vi "done(with var with tabs)subvi2backup.vi"(3 "error in (no error)":errorcluster, 5 "Image Src":T1) -> (0 "error out 2":errorcluster, 2 "Image Out 6":T1(plugin-control))   [LabVIEW 2011]
uses:
  <vilib>/vision/Image Controls.llb/IMAQ Image.ctl
  <vilib>/vision/NI_Vision_Development_Module.lvlib
panel:
  out "Image Dst Out":T1
  in  "Tab Control":T2(tab)
  out "Image Out 2":T1(plugin-control)
  out "Image Out 3":T1(plugin-control)
  out "Image Out 4":T1(plugin-control)
  out "Image Out 5":T1(plugin-control)
  out "Image Out 7":T1(plugin-control)
  in  "Parameters (OCR/OCV 1)":T3={"Threshold Mode"=1, "Fixed Threshold Range"={"Lower value"=1.0, "Upper value"=255.0}, "Advanced Threshold Data"={"Number of Blocks"=4, "Pixel Value Range"={"Lower value"=0, "Upper value"=255}, "Optimize For Speed"=FALSE, "Perform Bi-modal Calculation"=FALSE}, "Character Color"=0, "Reject Border"=FALSE, "Number Of Erosions"=0, "Size & Spacing"={"AutoSplit"=FALSE, "Min Bounding Rect Width"=160, "Max Bounding Rect Width"=200, "Min Bounding Rect Height"=200, "Max Bounding Rect Height"=240, "Min Character Size"=20, "Max Character Size"=65536, "Min Char Spacing"=1, "Max Horiz Element Spacing"=1, "Max Vert Element Spacing"=0}, "Read Options"={"Read Strategy"=1, "Read Resolution"=0, "Scale Dependant"=FALSE, "Aspect Ratio"=400, "Acceptance Level"=700, "Substitution Character"="?"}, "Valid Characters"=[], "Use Text Pattern"=FALSE, "Orientation"=0} {"Threshold Mode" items=["Fixed Range", "Uniform", "Linear", "Non Linear"]; "Character Color" items=["Dark on Light", "Light on Dark"]; "Read Options"."Read Strategy" items=["Aggressive", "Conservative"]; "Read Options"."Read Resolution" items=["Low", "Medium", "High"]; "Valid Characters"."Pre-defined characters" items=["Any Character", "User-defined Characters", "Alphabetic", "Alphanumeric", "Uppercase Letters", "Lowercase Letters", "Decimal Digits", "Hexadecimal Digits", "Pattern", "Force Space"]; "Orientation" items=["Baseline inside", "Baseline outside"]}
  in  "File Path (OCR/OCV 1)":path=path "D:/Program Files/National Instruments/Vision/OCR/CharacterSetFiles/OCRA30.abc"
  in  "ROI Descriptor (OCR/OCV 1)":T4={"Global Rectangle"=[390, 669, 561, 882], "Contours"=[{"ID"=enum."External", "Type"=3, "Coordinates"=[390, 669, 561, 882]}]} {"Contours"."Type" items=["No Selection", "Point", "Line", "Rectangle", "Oval", "Polygon", "Freehand Region", "Annulus", "Unused2", "Unused3", "Broken Line", "Freehand Line", "Rotated Rectangle"]}
  in  "Method (Filters 1)":T5(ring)=enum."Prewitt"
  in  "Niblack Deviation Factor (Threshold 1)":dbl=0.2
  in  "Kernel Size (Threshold 1)":cluster{"SizeX":i32, "SizeY":i32}={"SizeX"=32, "SizeY"=32}
  in  "Look For (Bright Objects) (Threshold 1)":u32(ring) items=["Bright Objects", "Dark Objects"]
  in  "Method (Threshold 1)":u32(ring)=1 items=["Niblack", "Background Correction"]
  in  "Color Plane (Color Plane Extraction 1)":i32(ring)=5 items=["Red", "Green", "Blue", "Hue", "Saturation", "Luminance", "Value", "Intensity"]
  out "String (OCR/OCV 1)":string
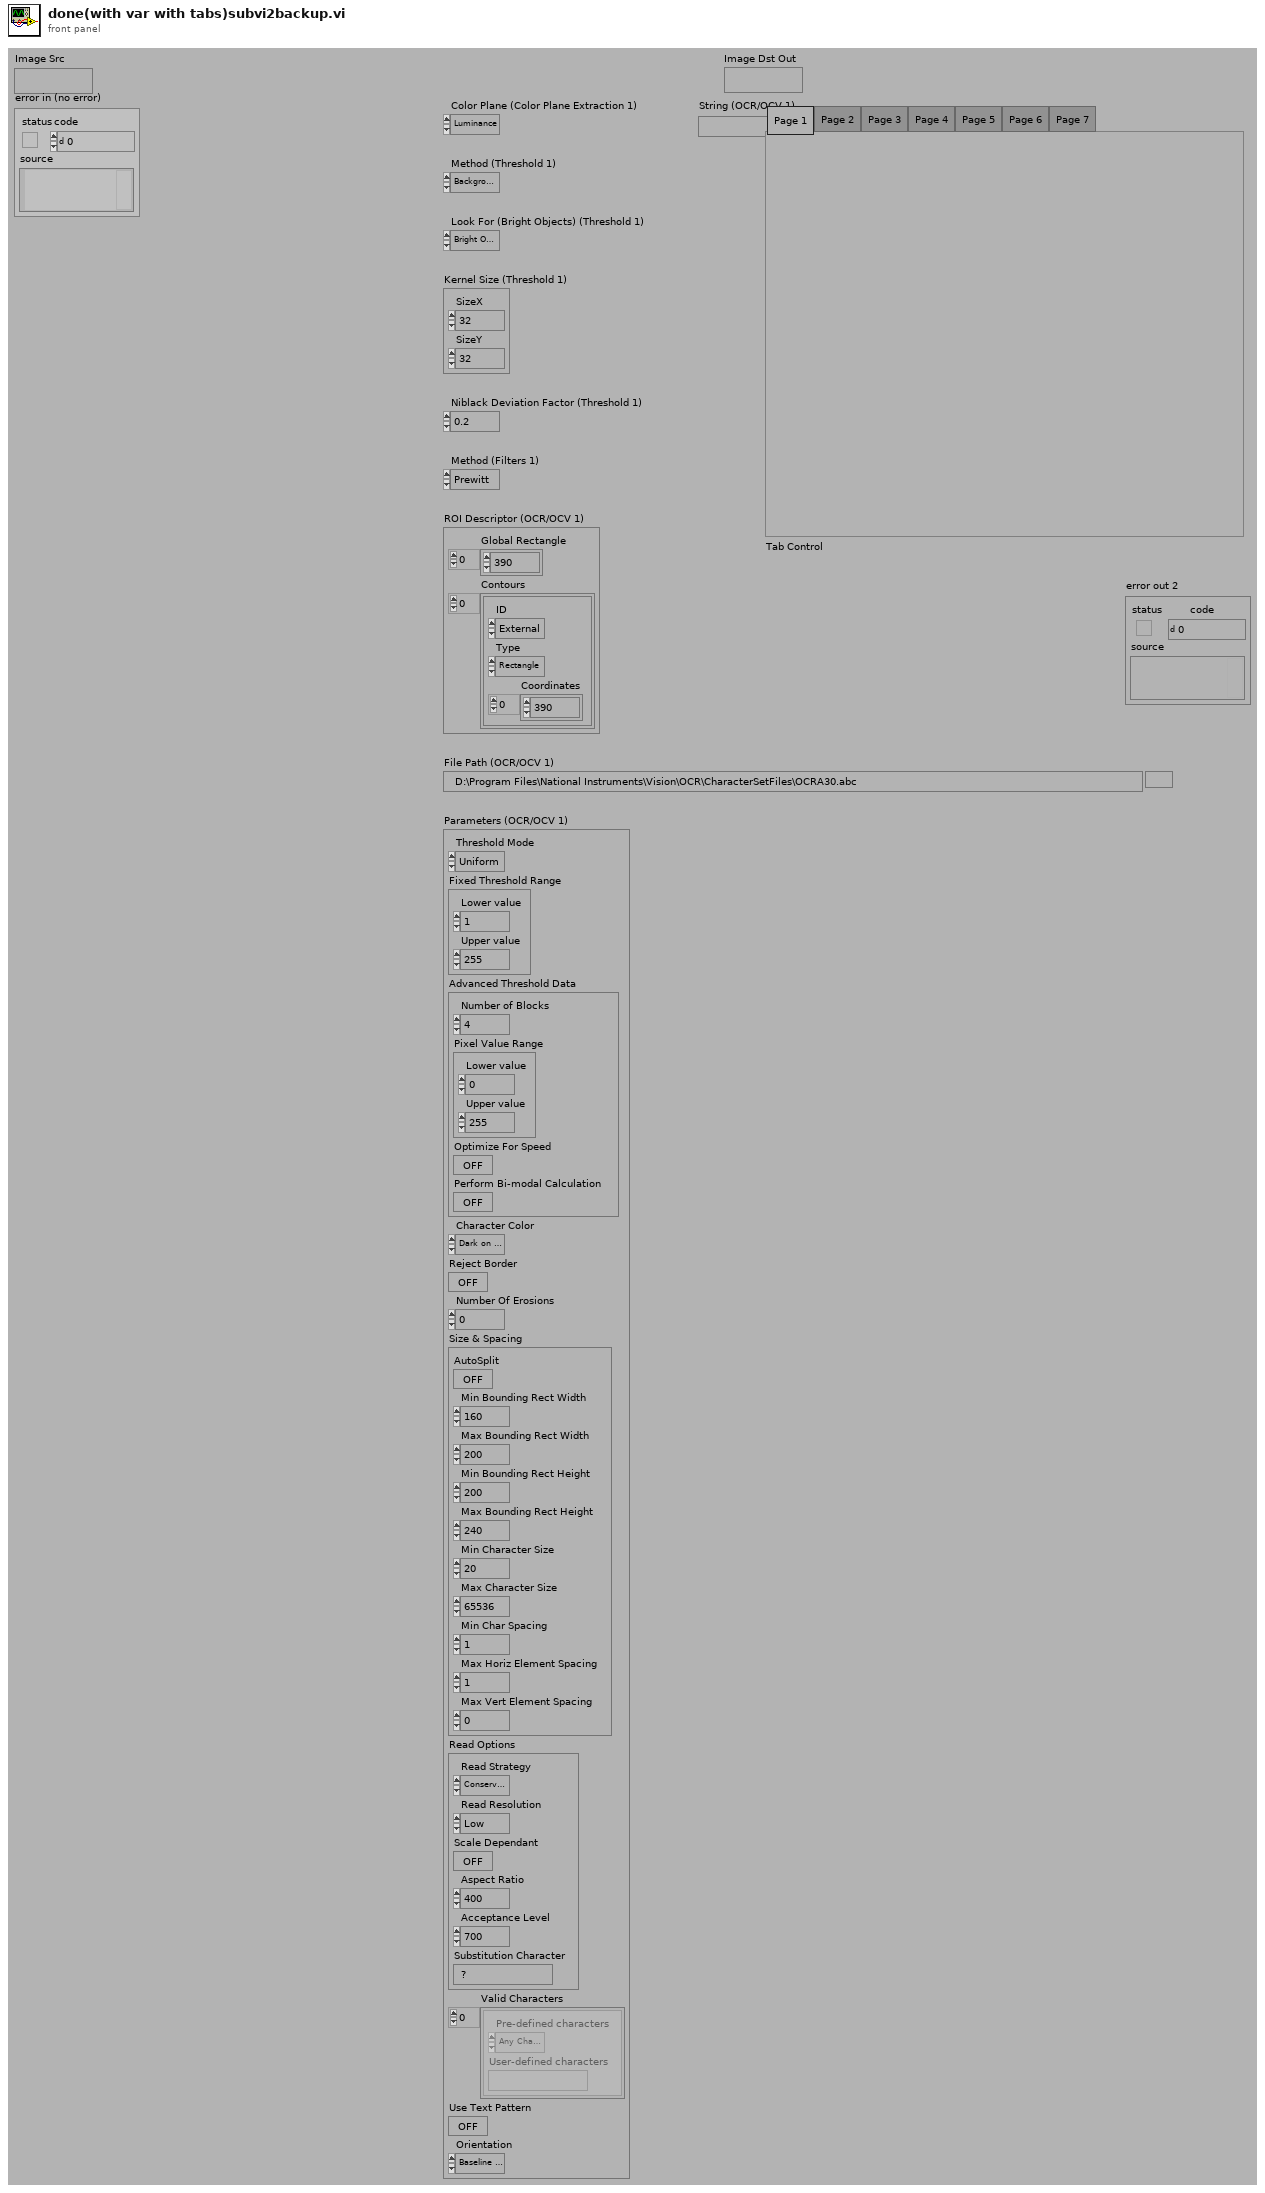
[diagram p1: front panel]
types:
  T1 = typedef "IMAQ Image.ctl" = refnum<image>
  T2 = enum32{"Page 1", "Page 2", "Page 3", "Page 4", "Page 5", "Page 6", "Page 7"}
  T3 = cluster{"Threshold Mode":i32, "Fixed Threshold Range":cluster{"Lower value":sgl, "Upper value":sgl}, "Advanced Threshold Data":cluster{"Number of Blocks":i32, "Pixel Value Range":cluster{"Lower value":i32, "Upper value":i32}, "Optimize For Speed":bool, "Perform Bi-modal Calculation":bool}, "Character Color":i32, "Reject Border":bool, "Number Of Erosions":i32, "Size & Spacing":cluster{"AutoSplit":bool, "Min Bounding Rect Width":i32, "Max Bounding Rect Width":i32, "Min Bounding Rect Height":i32, "Max Bounding Rect Height":i32, "Min Character Size":i32, "Max Character Size":i32, "Min Char Spacing":i32, "Max Horiz Element Spacing":i32, "Max Vert Element Spacing":i32}, "Read Options":cluster{"Read Strategy":i32, "Read Resolution":i32, "Scale Dependant":bool, "Aspect Ratio":i32, "Acceptance Level":i32, "Substitution Character":string}, "Valid Characters":cluster{"Pre-defined characters":i32, "User-defined characters":string}[], "Use Text Pattern":bool, "Orientation":u32}
  T4 = cluster{"Global Rectangle":i32[], "Contours":cluster{"ID":enum32{"External", "Internal"}, "Type":u32, "Coordinates":i32[]}[]}
  T5 = enum32{"Differentiation", "Gradient", "Prewitt", "Roberts", "Sigma", "Sobel"}
  T6 = cluster{"histogram":u32[], "Minimal Value":sgl, "Maximal Value":sgl, "Starting Value":sgl, "Interval Width":sgl, "Mean Value":sgl, "Standard  Variation":sgl, "Area (pixels)":i32}
  T7 = typedef "Image Type" = u32
  T8 = typedef "IMAQ OCR Session.ctl" = refnum<k1>
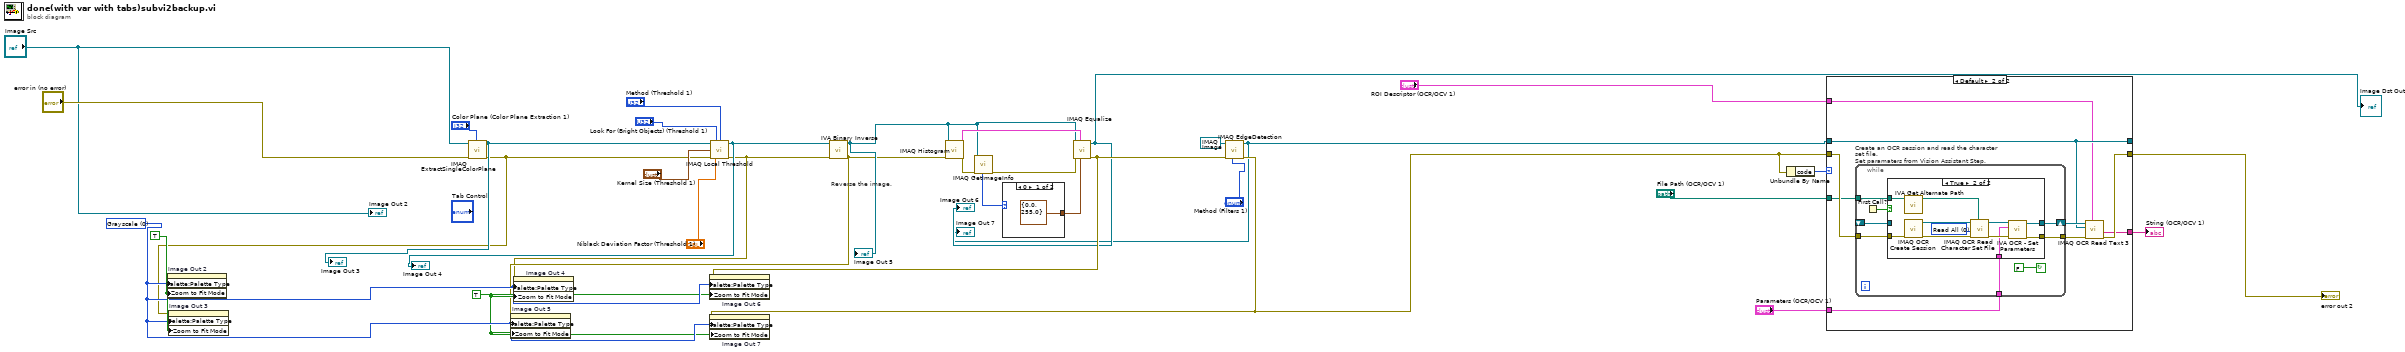
[diagram p0: block diagram]
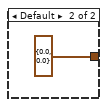
[diagram p4: hidden frame]
diagram:
  w16 = TRUE ("Zoom to Fit Mode")
  w18 = TRUE ("Zoom to Fit Mode")
  w17 = u32 0 items=["Grayscale", "Binary", "Gradient", "Rainbow", "Temperature", "User Defined"] ("Palette")
  # "Reverse the image."
  n1 = property on="Image Out 2" class="ImageControl"("Palette:Palette Type"=w17, "Zoom to Fit Mode"=w18) -> ()  [unwired: 2 in, 2 out]
  n2 = call "IMAQ ExtractSingleColorPlane"("Color Plane"="Color Plane (Color Plane Extraction 1)", "error in (no error)"="error in (no error)", "Image Src"="Image Src") -> ("error out"=w6:errorcluster, "Image Dst Out"=w14:T1)  [unwired: 1 in, 6 out]
  "Image Out 3" <- w14
  n3 = property on="Image Out 3" class="ImageControl"(error in=w6, "Palette:Palette Type"=w17, "Zoom to Fit Mode"=w18) -> ()  [unwired: 1 in, 2 out]
  n4 = call "IMAQ Local Threshold"("Image Src"=w14, "Look For (Bright Objects)"="Look For (Bright Objects) (Threshold 1)", "Method (Niblack)"="Method (Threshold 1)", "Window Size (32x32)"="Kernel Size (Threshold 1)", "error in (no error)"=w6, "Niblack Deviation Factor (0.2)"="Niblack Deviation Factor (Threshold 1)") -> ("Image Dst Out"=w13:T1, "error out"=w7:errorcluster)  [unwired: 2 in, 6 out]
  "Image Out 4" <- w13
  n5 = property on="Image Out 4" class="ImageControl"(error in=w7, "Palette:Palette Type"=w17, "Zoom to Fit Mode"=w16) -> ()  [unwired: 1 in, 2 out]
  n6 = call <vilib>:"IVA Binary Inverse.vi"("error in (no error)"=w7, "Image In"=w13) -> ("error out"=w8:errorcluster, "Image Out"=w12:T1)  [unwired: 8 out]
  "Image Out 5" <- w12
  n7 = property on="Image Out 5" class="ImageControl"(error in=w8, "Palette:Palette Type"=w17, "Zoom to Fit Mode"=w16) -> ()  [unwired: 1 in, 2 out]
  n8 = call "IMAQ Histogram"("error in (no error)"=w8, "Image"=w12) -> ("error out"=w15:errorcluster, "Histogram Report"=w28:T6)  [unwired: 3 in, 5 out]
  n9 = call "IMAQ GetImageInfo"("error in (no error)"=w15, "Image"=w12) -> ("error out"=w26:errorcluster, "Image Type"=w27:T7)  [unwired: 8 out]
  n10 = case shown="0" w27 {
    tunnel: [cluster{"Minimum":sgl, "Maximum":sgl} {"Minimum"=0.0, "Maximum"=255.0} ("Range") cluster{"Minimum":sgl, "Maximum":sgl} {"Minimum"=0.0, "Maximum"=0.0} ("Range")] -> w25
    frame 0 {
    }
    frame Default {
    }
  }
  n11 = call "IMAQ Equalize"("Range"=w25, "Histogram Report"=w28, "error in (no error)"=w26, "Image Src"=w12) -> ("error out"=w9:errorcluster, "Image Dst Out"=→"Image Out 6" →"Image Dst Out":T1)  [unwired: 2 in, 4 out]
  n12 = property on="Image Out 6" class="ImageControl"(error in=w9, "Palette:Palette Type"=w17, "Zoom to Fit Mode"=w16) -> ()  [unwired: 1 in, 2 out]
  n13 = call "IMAQ EdgeDetection"("Method"="Method (Filters 1)", "error in (no error)"=w9, "Image Src"=T1 refnum) -> ("error out"=w11:errorcluster, "Image Dst Out"=w3:T1)  [unwired: 3 in, 4 out]
  "Image Out 7" <- w3
  n14 = property on="Image Out 7" class="ImageControl"(error in=w11, "Palette:Palette Type"=w17, "Zoom to Fit Mode"=w16) -> ()  [unwired: 1 in, 2 out]
  n15 = Unbundle By Name(w11) -> ("code"=w19:i32)
  n16 = case shown="Default" w19 {
    tunnel: "File Path (OCR/OCV 1)" -> [_ w43]
    tunnel: w11 -> [_ w45]
    tunnel: w3 -> [w36 w40]
    tunnel: [_ w38] -> w10
    tunnel: [_ w37] -> w22
    tunnel: "Parameters (OCR/OCV 1)" -> [_ w44]
    tunnel: "ROI Descriptor (OCR/OCV 1)" -> [_ w39]
    tunnel: [w36 w40] -> _
    frame -1074396199, -1074396198 {
      # "Discard Coordinate System Error"
    }
    frame Default {
      n17 = while "Create an OCR session and read the character set file.\nSet paramaters from Vision Assistant Step." {
        shift-right: [w50] -> w41
        shift-left: _ -> [w49]
        tunnel: w45 -> [w52]
        tunnel: w44 -> [w48]
        tunnel: w43 -> [w47]
        tunnel: [w46] -> w42
        stop <- FALSE continue-if-true
        n18 = First Call?() -> (First Call?: T/F=w51:bool)
        n19 = case shown="True" w51 {
          tunnel: w47 -> [_ w57]
          tunnel: w52 -> [w54 w63]
          tunnel: [w55 w60] -> w50
          tunnel: [w54 w59] -> w46
          tunnel: w48 -> [_ w58]
          tunnel: w49 -> [w55 _]
          frame False {
          }
          frame True {
            w64 = 0 items=["Read All", "Read Character Set Only", "Read Properties Only"] ("Read Options")
            n20 = call <vilib>:"IVA Get Alternate Path.vi"("Path In"=w57) -> ("Path Out"=w56:path)  [unwired: 10 out]
            n21 = call "IMAQ OCR Create Session"("error in (no error)"=w63) -> ("error out"=w65:errorcluster, "IMAQ OCR Session"=w66:T8)  [unwired: 9 out]
            n22 = call "IMAQ OCR Read Character Set File"("File Path"=w56, "error in (no error)"=w65, "Read Options"=w64, "IMAQ OCR Session"=w66) -> ("error out"=w61:errorcluster, "IMAQ OCR Session (dup)"=w62:T8)  [unwired: 1 in, 5 out]
            n23 = call <vilib>:"IVA OCR - Set Parameters.vi"("error in (no error)"=w61, "Parameters"=w58, "IMAQ OCR Session"=w62) -> ("error out"=w59:errorcluster, "IMAQ OCR Session Out"=w60:T8)  [unwired: 7 out]
          }
        }
      }
      n24 = call "IMAQ OCR Read Text 3"("ROI Descriptor"=w39, "error in (no error)"=w42, "Image"=w40, "IMAQ OCR Session"=w41) -> ("error out"=w38:errorcluster, "Read String"=w37:string)  [unwired: 1 in, 5 out]
    }
  }
  "String (OCR/OCV 1)" <- w22
  "error out 2" <- w10
  "Image Out 2" <- "Image Src"
